vi "Color Classification.vi"() -> ()   [LabVIEW 2014]
doc: "This example shows how to use the classification VIs in NI Vision. Classification quickly identifies and classifies unknown objects in inspection images. First, use the Classification Training Interface to teach your application the types, or classes, of objects you want to classify. The Classification Training Interface creates a classifier file, which you then use to classify unknown objects into one of the classes you trained."
uses:
  <vilib>/vision/NI_Vision_Development_Module.lvlib
panel:
  in  "Stop":bool
  out "Image":T1(plugin-control)
  # "Overview: Demonstrates how to use the IMAQ Classify function with a color classifier file to classify the color within a Region of Interest (ROI).\nRequirements: Vision Development Software.\nInstructions:\n1. Run the VI.\n2. Draw a ROI in the image to see what class the color is associated with and the score. Hold down <Ctrl> to select more than one ROI."
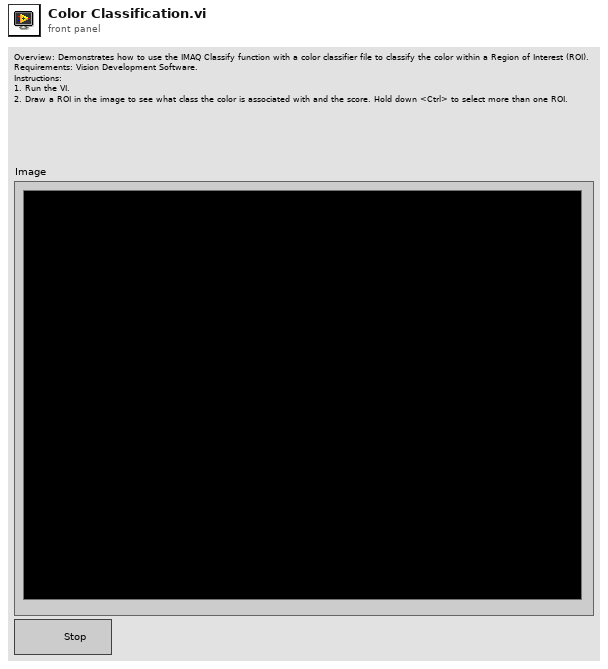
[diagram p1: front panel]
types:
  T1 = typedef "IMAQ Image.ctl" = refnum<image>
  T2 = typedef "IMAQ Rectangle" = cluster{"Left":i32, "Top":i32, "Right":i32, "Bottom":i32, "Rotation":dbl}
  T3 = typedef "Image Type" = u32
  T4 = typedef "ROI Descriptor" = cluster{"Global Rectangle":i32[], "Contours":cluster{"ID":enum32{"External", "Internal"}, "Type":u32, "Coordinates":i32[]}[]}
  T5 = typedef "IMAQ Classifier Session.ctl" = refnum<k1>
  T6 = cluster{"Desired Font (Application)":enum16{"User-specified Font", "Application Font", "System Font", "Dialog Font"}, "[User-specified Font]":cluster{"Font Name":string, "Size":i16, "Strikeout?":bool, "Italic?":bool, "Underline?":bool, "Outline?":bool, "Shadow?":bool, "Bold?":bool, "Rotation Angle":dbl}, "Horizontal Alignment":i16, "Vertical Alignment":i16}
  T7 = cluster{"Global Rectangle":i32[], "Contours":cluster{"Contour Type":u32, "ROI Type":u32, "Points":i32[]}[]}
  T8 = cluster{"Classification Score":sgl, "Identification Score":sgl}
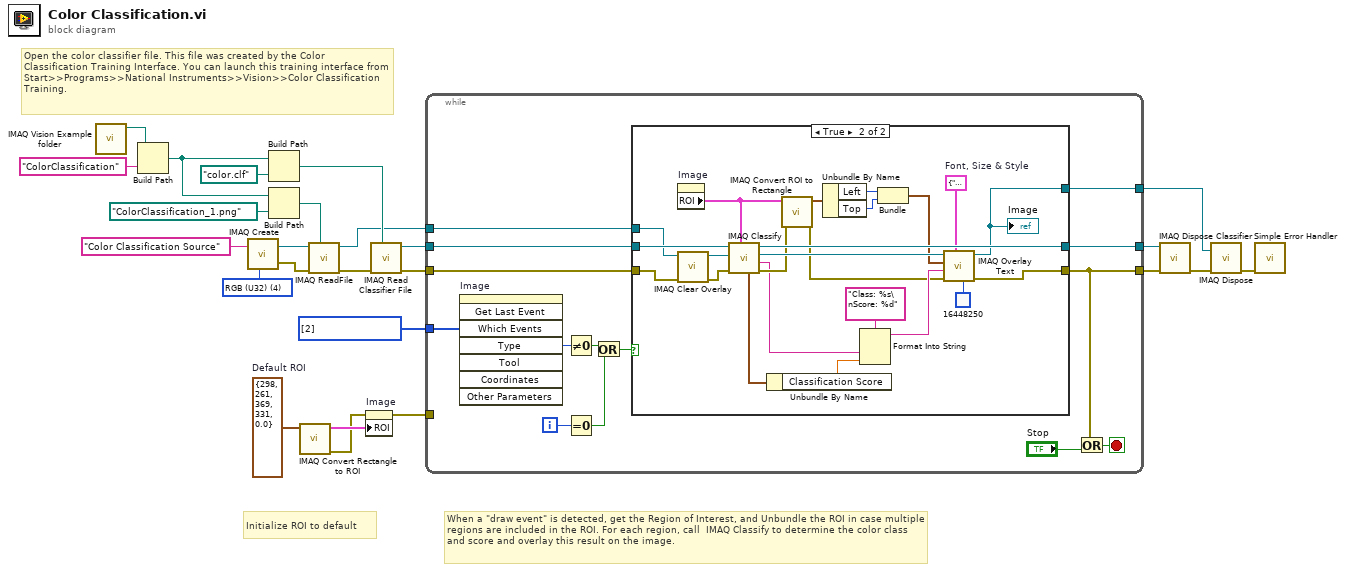
[diagram p0: block diagram]
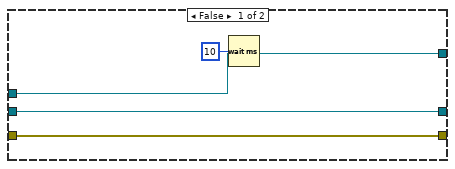
[diagram p2: hidden frame]
diagram:
  w3 = T2 {"Left"=298, "Top"=261, "Right"=369, "Bottom"=331, "Rotation"=0.0}  # Default ROI
  w7 = i32[] [2] items=["No Event"=0, "Click Event"=1, "Draw Event"=2, "Size Event"=4, "Scroll Event"=5, "Double Click Event"=8] ("Which Events")
  w23 = T3 4 items=["Grayscale (U8)", "Grayscale (I16)", "Grayscale (SGL)", "Complex (CSG)", "RGB (U32)", "HSL (U32)", "RGB (U64)", "Grayscale (U16)"] ("Image Type")
  # "Open the color classifier file. This file was created by the Color Classification Training Interface. You can launch this training interface from Start>>Programs>>National Instruments>>Vision>>Color Classification Training."
  # "Initialize ROI to default"
  # "When a \"draw event\" is detected, get the Region of Interest, and Unbundle the ROI in case multiple regions are included in the ROI. For each region, call  IMAQ Classify to determine the color class and score and overlay this result on the image."
  n1 = call "IMAQ Vision Example folder.vi"() -> ("Example Image Path"=w25:path)  [unwired: 11 in]
  n2 = Build Path(base path=w25, name or relative path="ColorClassification") -> (appended path=w20:path)
  n3 = call "IMAQ Create"("Image Name"="Color Classification Source", "Image Type"=w23) -> ("New Image"=w21:T1, "error out"=w5:errorcluster)  [unwired: 2 in, 1 out]
  n4 = Build Path(base path=w20, name or relative path=path "color.clf") -> (appended path=w17:path)
  n5 = Build Path(base path=w20, name or relative path=path "ColorClassification_1.png") -> (appended path=w18:path)
  n6 = call "IMAQ Convert Rectangle to ROI"("Rectangle"=w3) -> ("error out"=w1:errorcluster, "ROI Descriptor"=w2:T4)  [unwired: 8 in]
  n7 = call "IMAQ ReadFile"("File Path"=w18, "error in (no error)"=w5, "Image"=w21) -> ("error out"=w16:errorcluster, "Image Out"=w15:T1)  [unwired: 4 in, 3 out]
  n8 = property on="Image" class="ImageControl"(error in=w1, "ROI"=w2) -> (error out=w8:errorcluster)  [unwired: 1 in, 1 out]
  n9 = call "IMAQ Read Classifier File"("File Path"=w17, "error in (no error)"=w16) -> ("error out"=w13:errorcluster, "Classifier Session"=w14:T5)  [unwired: 2 in, 6 out]
  n10 = while {
    tunnel: w15 -> [w39]
    tunnel: w14 -> [w38]
    tunnel: w13 -> [w26]
    tunnel: [w37] -> w12
    tunnel: [w28] -> w10
    tunnel: [w36] -> w9
    tunnel: w8 -> [_]
    tunnel: w7 -> [w35]
    i -> [w32]
    stop <- w27 stop-if-true
    n11 = invoke on="Image" class="ImageControl" method="Get Last Event"("Which Events"=w35) -> ("Type"=w34:i32)  [unwired: 7 in, 7 out]
    n12 = Not Equal To 0?(x=w34) -> (x != 0?=w33:bool)
    n13 = Equal To 0?(x=w32) -> (x = 0?=w31:bool)
    n14 = Or(x=w33, y=w31) -> (x .or. y?=w30:bool)
    n15 = case shown="True" w30 {
      tunnel: w39 -> [w43 w61]
      tunnel: w38 -> [w42 w66]
      tunnel: w26 -> [w41 w63]
      tunnel: [w42 w65] -> w37
      tunnel: [w41 w64] -> w28
      tunnel: [w43 w45] -> w36
      frame False {
        n16 = Wait (ms)(milliseconds to wait=u32 10) -> ()  [unwired: 1 out]
      }
      frame True {
        w51 = T6 {"Desired Font (Application)"=enum."Application Font", "[User-specified Font]"={"Font Name"="", "Size"=12, "Strikeout?"=FALSE, "Italic?"=FALSE, "Underline?"=FALSE, "Outline?"=FALSE, "Shadow?"=FALSE, "Bold?"=FALSE, "Rotation Angle"=0.0}, "Horizontal Alignment"=0, "Vertical Alignment"=1}  # Font, Size & Style
        n17 = property on="Image" class="ImageControl"() -> ("ROI"=w47:T7)  [unwired: 2 in, 2 out]
        n18 = call "IMAQ Clear Overlay"("error in (no error)"=w63, "Image"=w61) -> ("error out"=w62:errorcluster, "Image Out"=w60:T1)  [unwired: 8 in]
        n19 = call "IMAQ Classify"("ROI Descriptor"=w47, "error in (no error)"=w62, "Image"=w60, "Classifier Session"=w66) -> ("error out"=w49:errorcluster, "Class"=w44:string, "Image (dup)"=w56:T1, "Classifier Session (dup)"=w65:T5, "Scores"=w57:T8)  [unwired: 3 out]
        n20 = Unbundle By Name(w57) -> ("Classification Score"=w58:sgl)
        n21 = call "IMAQ Convert ROI to Rectangle"("error in (no error)"=w49, "ROI Descriptor"=w47) -> ("error out"=w48:errorcluster, "Rectangle"=w55:T2)  [unwired: 7 in]
        n22 = Unbundle By Name(w55) -> ("Left"=w50:i32, "Top"=w54:i32)
        n23 = Format Into String(format string="Class: %s\nScore: %d" ("string"), w44, w58) -> (resulting string=w52:string)  [unwired: 2 in, 1 out]
        n24 = Bundle("Left"=w50, "Top"=w54) -> (w53:cluster{"Left":i32, "Top":i32})  [unwired: 1 in]
        n25 = call "IMAQ Overlay Text"("BG Color (Transparent)"=u32 16448250, "Font, Size & Style"=w51, "error in (no error)"=w48, "String"=w52, "Origin"=w53, "Image"=w56) -> ("error out"=w64:errorcluster, "Image Out"=w45:T1)  [unwired: 4 in]
        "Image" <- w45
      }
    }
    n26 = Or(x=w28, y="Stop") -> (x .or. y?=w27:bool)
  }
  n27 = call "IMAQ Dispose Classifier"("error in (no error)"=w10, "Classifier Session"=w12) -> ("error out"=w11:errorcluster)  [unwired: 9 out]
  n28 = call "IMAQ Dispose"("Image"=w9, "error in (no error)"=w11) -> ("error out"=w6:errorcluster)  [unwired: 4 in]
  n29 = call <vilib>:"Simple Error Handler.vi"("error in (no error)"=w6) -> ()  [unwired: 1 in, 8 out]
